vi "InitCamera.vi"(3 "Frame Grabber Settings":T4={"Name"="", "Digitizer"=2, "Input"=1, "Width"=320, "Height"=240, "Input format"=enum."NTSC", "Frame rate"=0.0, "Reserved"=0, "Dialogs"=0} {"Frame rate" format="%#1_6g"; "Dialogs" format="%.0b"}) -> (0 "error out":errorcluster={"status"=TRUE, "code"=-43, "source"=""}, 1 "QT Ref Out":T2)   [LabVIEW 2024]
doc: "This VI initializes the camera. Multiple cameras can be used and identified by altering the camera input. By changing the poly option, the user can switch between NTSC, PAL, and Advanced settings.\n\nSee the LiveFeed “behavior” in the behaviors palette for a quick sample live camera feed program."
uses:
  <userlib>/ImageProcessing/QTLIB_2595_LV86/QT_Private.ctl
  <userlib>/ImageProcessing/QTLIB_2595_LV86/QT_Compression.ctl
  <userlib>/ImageProcessing/QTLIB_2595_LV86/QT_FrameGrabber.ctl
  <userlib>/ImageProcessing/QTLIB_2595_LV86/QT_Ref.ctl
  <userlib>/ImageProcessing/QTLIB_2595_LV86/QT_Video.ctl
panel:
  in  "Video Settings in":T1 {"Dialogs" format="%.0b"; "Color format" items=["Black & White (8 bits)", "RGB (24 bits)", "RGBx (32 bits)", "RGBA (32bits)", "RGB B&W (32 bits)", "HSI (24 bits)", "HSIx (32 bits)", "HSI B&W (32 bits)"]; "Brightness" format="%.2f"; "Contrast" format="%.2f"; "Sharpness" format="%.2f"; "Black Level" format="%.2f"; "White Level" format="%.2f"; "Saturation" format="%.2f"; "Hue" format="%.2f"}
  in  "Compression":i32(slide)=745 scale=0.0..1024.0 scale format="%x"
  in  "Codec (raw )":T3(ring)=enum."jpeg"
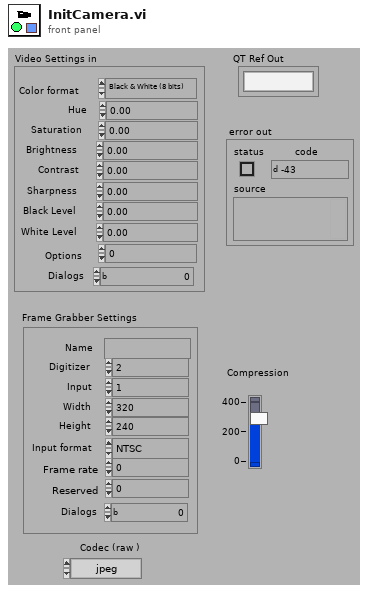
[diagram p1: front panel]
types:
  T1 = typedef "QT_Video.ctl" = cluster{"Color format":u32, "Hue":dbl, "Saturation":dbl, "Brightness":dbl, "Contrast":dbl, "Sharpness":dbl, "Black Level":dbl, "White Level":dbl, "Options":i32, "Dialogs":u32}
  T2 = typedef "QT_Ref.ctl" = refnum<k1>
  T3 = enum16{"rle ", "WRLE", "cvid", "yuv2", "dvcp", "dvc ", "dvpp", "smc ", "h261", "h263", "mjp2", "mjpa", "mjpb", "mp4v", "raw ", "VP31", "jpeg", "8BPS", "png ", "SVQ1", "SVQ3", "tga ", "tiff", "rpza", "ZyGo"}
  T4 = typedef "QT_FrameGrabber.ctl" = cluster{"Name":string, "Digitizer":i32, "Input":i32, "Width":i32, "Height":i32, "Input format":enum32{"NTSC", "PAL", "Secam"}, "Frame rate":dbl, "Reserved":i32, "Dialogs":u32}
  T5 = typedef "QT_Compression.ctl" = cluster{"Compression":i32, "Format":i32, "Codec":i32, "Comp. Quality":i32, "Key Frame":i32, "Dialogs":u32}
  T6 = typedef "QT_Private.ctl" = cluster{"reserved 1":i32, "reserved 2":i32, "reserved 3":i32, "reserved 4":i32}
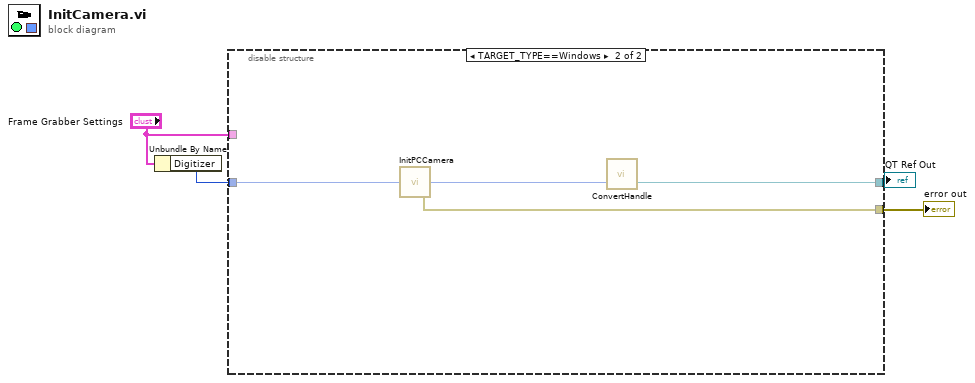
[diagram p0: block diagram]
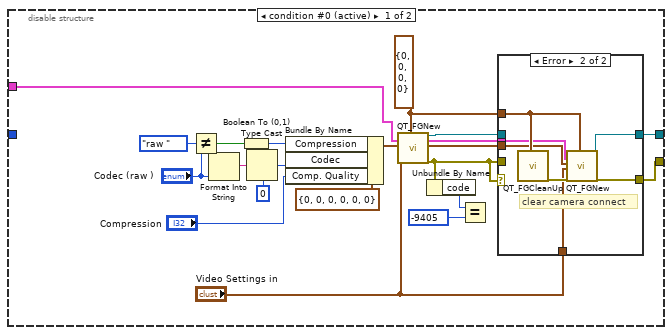
[diagram p2: hidden frame]
diagram:
  n1 = Unbundle By Name("Frame Grabber Settings") -> ("Digitizer"=w1:i32)
  n2 = disable-structure shown="TARGET_TYPE==Windows" {
    disable-tunnel: [w11 w35] -> w4
    disable-tunnel: [w9 w33] -> w3
    disable-tunnel: w1 -> [_ w36]
    disable-tunnel: "Frame Grabber Settings" -> [w5 _]
    frame condition #0 (active) {
      w12 = T6 {"reserved 1"=0, "reserved 2"=0, "reserved 3"=0, "reserved 4"=0} ("Private")
      n3 = Not Equal?(x=T3."raw " ("codec (raw )"), y="Codec (raw )") -> (x != y?=w16:bool)
      n4 = Format Into String("Codec (raw )") -> (resulting string=w23:string)  [unwired: 3 in, 1 out]
      n5 = Boolean To (0,1)(Boolean=w16) -> (0, 1=w15:i16)
      n6 = Type Cast(type=0 ("Codec"), x=w23) -> (*(type *) &x=w22:i32)
      n7 = Bundle By Name(cluster=T5 {"Compression"=0, "Format"=0, "Codec"=0, "Comp. Quality"=0, "Key Frame"=0, "Dialogs"=0} ("Compression Settings"), "Compression"=w15, "Codec"=w22, "Comp. Quality"="Compression") -> (w10:T5)
      n8 = call <userlib>:"QT_FGNew.vi"("Frame Grabber Settings"=w5, "Compression Settings"=w10, "Video Settings in"="Video Settings in", "Private"=w12) -> ("QT Ref Out"=w7:T2, "error out"=w6:errorcluster)  [unwired: 1 in, 13 out]
      n9 = Unbundle By Name(w6) -> ("code"=w14:i32)
      n10 = Equal?(x=w14, y=-9405) -> ()  [unwired: 1 out]
      n11 = case shown="Error" w6 {
        tunnel: w12 -> [_ w31]
        tunnel: [w25 w30] -> w11
        tunnel: w6 -> [w25 _]
        tunnel: w5 -> [_ w29]
        tunnel: w10 -> [_ w28]
        tunnel: [w24 w27] -> w9
        tunnel: "Video Settings in" -> [_ w26]
        tunnel: w7 -> [w24 _]
        frame No Error {
        }
        frame Error {
          # "clear camera connect"
          n12 = call <userlib>:"QT_FGCleanUp.vi"("Private"=w31) -> ("error out"=w32:errorcluster)  [unwired: 18 in]
          n13 = call <userlib>:"QT_FGNew.vi"("Frame Grabber Settings"=w29, "Compression Settings"=w28, "Video Settings in"=w26, "error in (no error)"=w32, "Private"=w31) -> ("QT Ref Out"=w27:T2, "error out"=w30:errorcluster)  [unwired: 13 out]
        }
      }
    }
    frame condition #1 {
      n14 = call <vilib>:"InitPCCamera.vi"("index"=w36) -> ("error out"=w35:errorcluster, "cameraReference"=w34:i64)  [unwired: 1 out]
      n15 = call <vilib>:"ConvertHandle.vi"("Camera Reference In"=w34) -> ("QT Ref Out"=w33:T2)  [unwired: 1 in, 1 out]
    }
  }
  "error out" <- w4
  "QT Ref Out" <- w3
